vi "loop_while.vi"() -> ()   [LabVIEW 2019]
panel:
  in  "condition":i32
  out "Numeric":i32
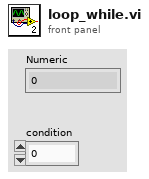
[diagram p1: front panel]
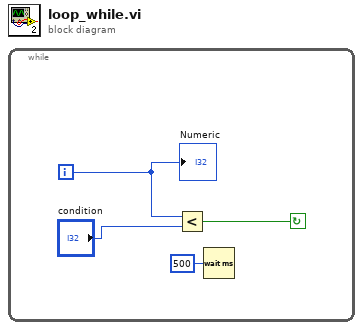
[diagram p0: block diagram]
diagram:
  n1 = while {
    i -> [w4]
    stop <- w3 continue-if-true
    n2 = Less?(x=w4, y="condition") -> (x < y?=w3:bool)
    n3 = Wait (ms)(milliseconds to wait=u32 500) -> ()  [unwired: 1 out]
    "Numeric" <- w4
  }
